vi "1,3A PWM MotorControl and VBattSense.vi"() -> ()   [LabVIEW 2011]
doc: "This VI is te Main VI to control the motors and the sense the Battery Voltage.\nMOTORS:\n\nThe motors are limited to given ranges in the setpoint VI. In general, there are two different servos that have to be actuated:\nThe Sailwinch has to work in its full range. The max range of the inout is form 0 to 1. The conversion to PW times is perfromed in Step 2 (In-VI documentation). The maximum range of this Servo was experimentally determined.\nThe Rudder Servo is limited to certain angles. The range of the rudder is determined through the control Rudder Range. The values will be modified by the Rudder Trim control, which allows the user to set a neutral rudder position. \nThe outputs of the Motor control are PWM signal times in us, which are sent to the FPGA VI."
uses:
  2-Think/2 Typedefs/rudder angle.ctl
  2-Think/2 Typedefs/sail setpt.ctl
  <vilib>/rvi/interface/nirviOpenFPGA/nirviOpenFPGA.xnode
  <vilib>/rvi/interface/nirviCloseFPGA/nirviCloseFPGA.xnode
  <vilib>/rvi/interface/nirviReadWriteControl/nirviReadWriteControl.xnode
  2-Think/2 Globals/2 Global.vi
  FPGA Bitfiles/SailBot_FPGATarget3_3APWMMotorContro_A9AA4CC4.lvbitx
  FPGA/1,3A PWM-MotorControl and VBattSense FPGA.vi
  FPGA Bitfiles/SailBot_FPGATarget_1,3APWM-MotorCon_F493B744.lvbitx
panel:
  in  "min winch duty (us)":u32=1130
  in  "max winch duty (us)":u32=1920
  in  "winch percentage min":T1
  in  "winch percentage max":T1=1.0
  in  "Reverse Winch Direction":bool=TRUE
  in  "# samples to average":u16=1500
  out "Averaged VBatt bitstring":bool[](array[boolean])
  out "vBatt":dbl
  out "vBatt from FPGA\n(unscaled)":u16
  in  "Rudder Range":dbl=80.0
  in  "Rudder Trim":dbl(slide) scale=-20.0..20.0
  out "Sail Position":T1
  out "Rudder Angle":T2
  out "error out":errorcluster
  # "with LSB disabled,\nuncertainty is +-0.08V"
  # "LSB disabled\n(plugged in to \nreserved pin \naccidentally)"
  # "LSB"
  # "MSB"
  # "these two will limit\nthe winch movement to\na percentage of its\nknown range, as a quick fix"
  # "these #s set the \nendpoints independently\nof the percentages\nabove. A better long-term\nsolution than the %s"
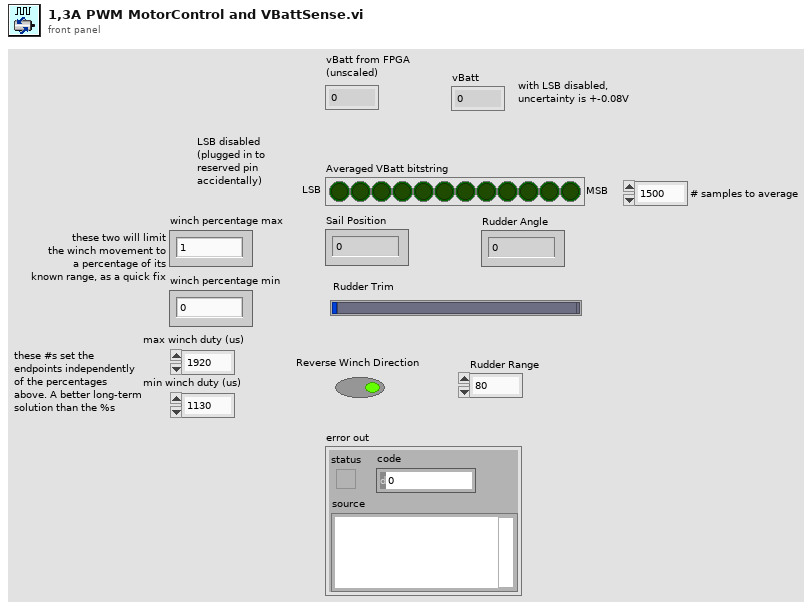
[diagram p1: front panel]
types:
  T1 = typedef "sail setpt.ctl" = dbl
  T2 = typedef "rudder angle.ctl" = dbl
  T3 = typedef "setpoints to boat.ctl" = cluster{"Sail Position":T1, "Rudder Angle":T2}
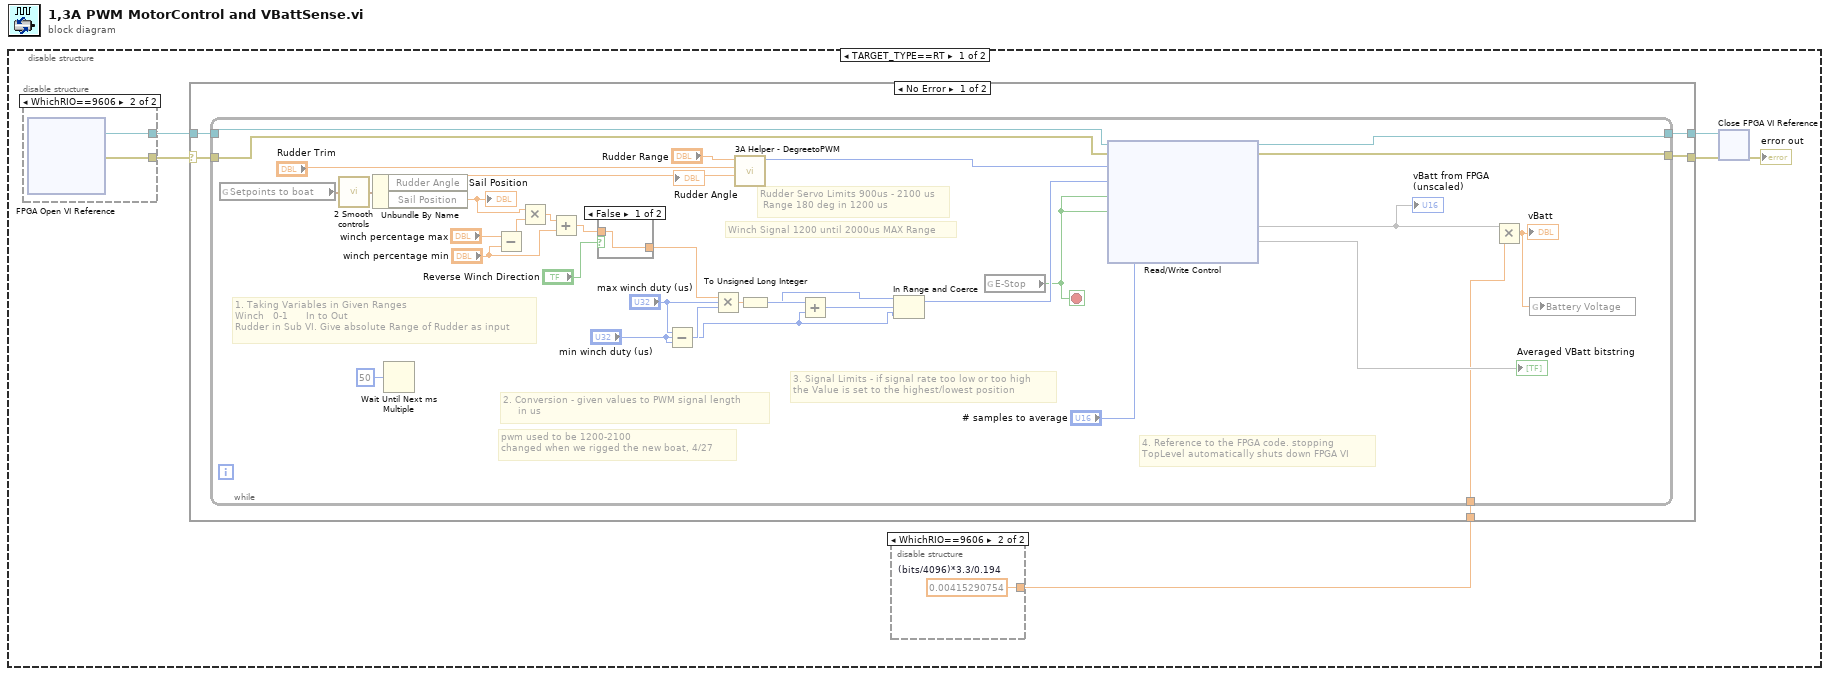
[diagram p0: block diagram]
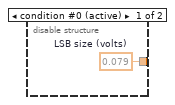
[diagram p2: hidden frame]
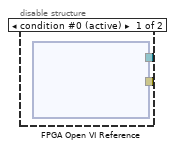
[diagram p3: hidden frame]
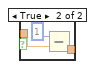
[diagram p4: hidden frame]
diagram:
  n1 = disable-structure shown="TARGET_TYPE==RT" {
    frame condition #0 {
      n2 = disable-structure shown="WhichRIO==9606" {
        disable-tunnel: [w9 w11] -> w5
        disable-tunnel: [w10 w12] -> w4
        frame condition #0 (active) {
          n3 = xnode "FPGA Open VI Reference"() -> ("FPGA VI Reference Out"=w9:refnum<k20>, "error out"=w10:errorcluster)  [unwired: 2 in]
        }
        frame condition #1 {
          n4 = xnode "FPGA Open VI Reference"() -> ("FPGA VI Reference Out"=w11:refnum<k20>, "error out"=w12:errorcluster)  [unwired: 2 in]
        }
      }
      n5 = disable-structure shown="WhichRIO==9606" {
        disable-tunnel: [w7 w8] -> w1
        frame condition #0 (active) {
          w7 = 0.079  # LSB size (volts)
        }
        frame condition #1 {
          w8 = 0.00415290754  # (bits/4096)*3.3/0.194
        }
      }
      n6 = case shown="No Error" w4 {
        selector: w4 -> [w17 w54]
        tunnel: [w14 w55] -> w3
        tunnel: [w15 w54] -> w2
        tunnel: w5 -> [w16 w55]
        tunnel: w1 -> [w13 _]
        frame No Error {
          n7 = while {
            tunnel: w16 -> [w46]
            tunnel: w17 -> [w47]
            tunnel: [w45] -> w15
            tunnel: [w44] -> w14
            tunnel: w13 -> [w32]
            stop <- w37 stop-if-true
            # "pwm used to be 1200-2100\nchanged when we rigged the new boat, 4/27"
            # "Rudder Servo Limits 900us - 2100 us\n Range 180 deg in 1200 us"
            # "1. Taking Variables in Given Ranges\nWinch   0-1      In to Out\nRudder in Sub VI. Give absolute Range of Rudder as input"
            # "2. Conversion - given values to PWM signal length\n     in us"
            # "3. Signal Limits - if signal rate too low or too high \nthe Value is set to the highest/lowest position"
            # "4. Reference to the FPGA code. stopping \nTopLevel automatically shuts down FPGA VI"
            # "Winch Signal 1200 until 2000us MAX Range"
            n8 = global read "2 Global.vi" "Setpoints to boat"() -> (w29:T3)
            n9 = call "2 Smooth controls.vi"("Setpoints in"=w29) -> ("Smoothed Setpoints out"=w28:T3)  [unwired: 4 in]
            n10 = Unbundle By Name(w28) -> ("Rudder Angle"=w30:T2, "Sail Position"=w18:T1)
            "Rudder Angle" <- w30
            "Sail Position" <- w18
            n11 = Wait Until Next ms Multiple(millisecond multiple=u32 50) -> ()  [unwired: 1 out]
            n12 = Subtract(x="winch percentage max", y="winch percentage min") -> (x-y=w21:T1)
            n13 = Multiply(x=w18, y=w21) -> (x*y=w19:T1)
            n14 = Add(x=w19, y="winch percentage min") -> (x+y=w20:T1)
            n15 = case shown="False" "Reverse Winch Direction" {
              tunnel: [w50 w52] -> w24
              tunnel: w20 -> [w50 w51]
              frame False {
              }
              frame True {
                n16 = Subtract(x=1, y=w51) -> (x-y=w52:T1)
              }
            }
            n17 = Subtract(x="max winch duty (us)", y="min winch duty (us)") -> (x-y=w27:u32)
            n18 = Multiply(x=w24, y=w27) -> (x*y=w49:T1)
            n19 = call "3A Helper - DegreetoPWM.vi"("Rudder Angle"=w30, "Rudder Trim"="Rudder Trim", "Rudder Range (deg)"="Rudder Range") -> ("Servo Position (us)"=w42:u32)  [unwired: 8 in]
            n20 = To Unsigned Long Integer(number=w49) -> (unsigned 32bit integer=w48:u32)
            n21 = Add(x=w48, y="min winch duty (us)") -> (x+y=w41:u32)
            n22 = In Range and Coerce(upper limit="max winch duty (us)", x=w41, lower limit="min winch duty (us)") -> (coerced(x)=w40:u32)  [unwired: 1 out]
            n23 = global read "2 Global.vi" "E-Stop"() -> (w37:bool)
            n24 = xnode "Read/Write Control"("FPGA VI Reference In"=w46, "error in"=w47, "Rudder Duty (uSec)"=w42, "Winch Duty (uSec)"=w40, "stop PWM"=w37, "stop VBatt Sense"=w37, "VBatt samples to average"="# samples to average") -> ("FPGA VI Reference Out"=w44:refnum<k20>, "error out"=w45:errorcluster, "vBatt ADC bits"=w36, "Averaged bitstring"=→"Averaged VBatt bitstring")
            "vBatt from FPGA\n(unscaled)" <- w36
            n25 = Multiply(x=w36, y=w32) -> (x*y=w35:dbl)
            "vBatt" <- w35
            n26 = global write "2 Global.vi" "Battery Voltage"(w35) -> ()
          }
        }
        frame Error {
          # "Error occurred. Do not run."
        }
      }
      n27 = xnode "Close FPGA VI Reference"("FPGA VI Reference In"=w3, "error in"=w2) -> ("error out"=→"error out":errorcluster)
    }
    frame condition #1 (active) {
    }
  }
